vi "SixWheelDriveTrainControl.vi"(0 "dead_or_alive":bool, 1 "Change to Open Loop":bool, 2 "Becky":T1={"DeviceStatus"={"status"=FALSE, "code"=0, "source"=""}, "Type"=enum."PWM", "PWM"={"Digital Module"=enum."Digital Module 1", "PWM Channel"=enum."Invalid", "DeadBand"={"Name"="", "maxPositivePwm"=0, "minPositivePwm"=0, "centerPwm"=0, "maxNegativePwm"=0, "minNegativePwm"=0, "angularRange"=0}}, "CAN"={"Device Number"=0, "Control Mode"=enum."Percent VBus", "Semaphore"=refnum, "Max Vout"=12.0}, "Invert"=FALSE, "TransformRef"=refnum, "InvTransformRef"=refnum}, 3 "Brian":T1={"DeviceStatus"={"status"=FALSE, "code"=0, "source"=""}, "Type"=enum."PWM", "PWM"={"Digital Module"=enum."Digital Module 1", "PWM Channel"=enum."Invalid", "DeadBand"={"Name"="", "maxPositivePwm"=0, "minPositivePwm"=0, "centerPwm"=0, "maxNegativePwm"=0, "minNegativePwm"=0, "angularRange"=0}}, "CAN"={"Device Number"=0, "Control Mode"=enum."Percent VBus", "Semaphore"=refnum, "Max Vout"=12.0}, "Invert"=FALSE, "TransformRef"=refnum, "InvTransformRef"=refnum}, 4 "Curt":T1={"DeviceStatus"={"status"=FALSE, "code"=0, "source"=""}, "Type"=enum."PWM", "PWM"={"Digital Module"=enum."Digital Module 1", "PWM Channel"=enum."Invalid", "DeadBand"={"Name"="", "maxPositivePwm"=0, "minPositivePwm"=0, "centerPwm"=0, "maxNegativePwm"=0, "minNegativePwm"=0, "angularRange"=0}}, "CAN"={"Device Number"=0, "Control Mode"=enum."Percent VBus", "Semaphore"=refnum, "Max Vout"=12.0}, "Invert"=FALSE, "TransformRef"=refnum, "InvTransformRef"=refnum}, 5 "Owen":T1={"DeviceStatus"={"status"=FALSE, "code"=0, "source"=""}, "Type"=enum."PWM", "PWM"={"Digital Module"=enum."Digital Module 1", "PWM Channel"=enum."Invalid", "DeadBand"={"Name"="", "maxPositivePwm"=0, "minPositivePwm"=0, "centerPwm"=0, "maxNegativePwm"=0, "minNegativePwm"=0, "angularRange"=0}}, "CAN"={"Device Number"=0, "Control Mode"=enum."Percent VBus", "Semaphore"=refnum, "Max Vout"=12.0}, "Invert"=FALSE, "TransformRef"=refnum, "InvTransformRef"=refnum}, 6 "CaseVar":i32, 8 "x axis value":dbl, 10 "y axis value":dbl) -> (7 "CaseVarReturn":i32, 9 "x axis value 2":dbl, 11 "y axis value 2":dbl, 16 "BeckyOutput":T1={"DeviceStatus"={"status"=FALSE, "code"=0, "source"=""}, "Type"=enum."PWM", "PWM"={"Digital Module"=enum."Digital Module 1", "PWM Channel"=enum."Invalid", "DeadBand"={"Name"="", "maxPositivePwm"=0, "minPositivePwm"=0, "centerPwm"=0, "maxNegativePwm"=0, "minNegativePwm"=0, "angularRange"=0}}, "CAN"={"Device Number"=0, "Control Mode"=enum."Percent VBus", "Semaphore"=refnum, "Max Vout"=12.0}, "Invert"=FALSE, "TransformRef"=refnum, "InvTransformRef"=refnum}, 17 "BrianOutput":T1={"DeviceStatus"={"status"=FALSE, "code"=0, "source"=""}, "Type"=enum."PWM", "PWM"={"Digital Module"=enum."Digital Module 1", "PWM Channel"=enum."Invalid", "DeadBand"={"Name"="", "maxPositivePwm"=0, "minPositivePwm"=0, "centerPwm"=0, "maxNegativePwm"=0, "minNegativePwm"=0, "angularRange"=0}}, "CAN"={"Device Number"=0, "Control Mode"=enum."Percent VBus", "Semaphore"=refnum, "Max Vout"=12.0}, "Invert"=FALSE, "TransformRef"=refnum, "InvTransformRef"=refnum}, 18 "CurtOutput":T1={"DeviceStatus"={"status"=FALSE, "code"=0, "source"=""}, "Type"=enum."PWM", "PWM"={"Digital Module"=enum."Digital Module 1", "PWM Channel"=enum."Invalid", "DeadBand"={"Name"="", "maxPositivePwm"=0, "minPositivePwm"=0, "centerPwm"=0, "maxNegativePwm"=0, "minNegativePwm"=0, "angularRange"=0}}, "CAN"={"Device Number"=0, "Control Mode"=enum."Percent VBus", "Semaphore"=refnum, "Max Vout"=12.0}, "Invert"=FALSE, "TransformRef"=refnum, "InvTransformRef"=refnum}, 19 "OwenOutput":T1={"DeviceStatus"={"status"=FALSE, "code"=0, "source"=""}, "Type"=enum."PWM", "PWM"={"Digital Module"=enum."Digital Module 1", "PWM Channel"=enum."Invalid", "DeadBand"={"Name"="", "maxPositivePwm"=0, "minPositivePwm"=0, "centerPwm"=0, "maxNegativePwm"=0, "minNegativePwm"=0, "angularRange"=0}}, "CAN"={"Device Number"=0, "Control Mode"=enum."Percent VBus", "Semaphore"=refnum, "Max Vout"=12.0}, "Invert"=FALSE, "TransformRef"=refnum, "InvTransformRef"=refnum})   [LabVIEW 2012]
uses:
  <vilib>/Rock Robotics/WPI/MotorControl/WPI_MotorControlDeviceRef.ctl
  <vilib>/Rock Robotics/SystemInterfaces/Typedef/FPGA_TypedefDigitalModule.ctl
  <vilib>/Rock Robotics/SystemInterfaces/DIO/FPGA_DIOPWMChannel.ctl
  <vilib>/Rock Robotics/WPI/PWM/WPI_PWMDeadband.ctl
  <vilib>/Rock Robotics/WPI/CAN/Jaguar/SubVIs/WPI_CANJaguar_ControlMode.ctl
  <vilib>/Rock Robotics/WPI/PWM/WPI_PWMTransform_ConPane.ctl
  <vilib>/Rock Robotics/WPI/CAN/Jaguar/SubVIs/WPI_CANJaguar_SpeedReference.ctl
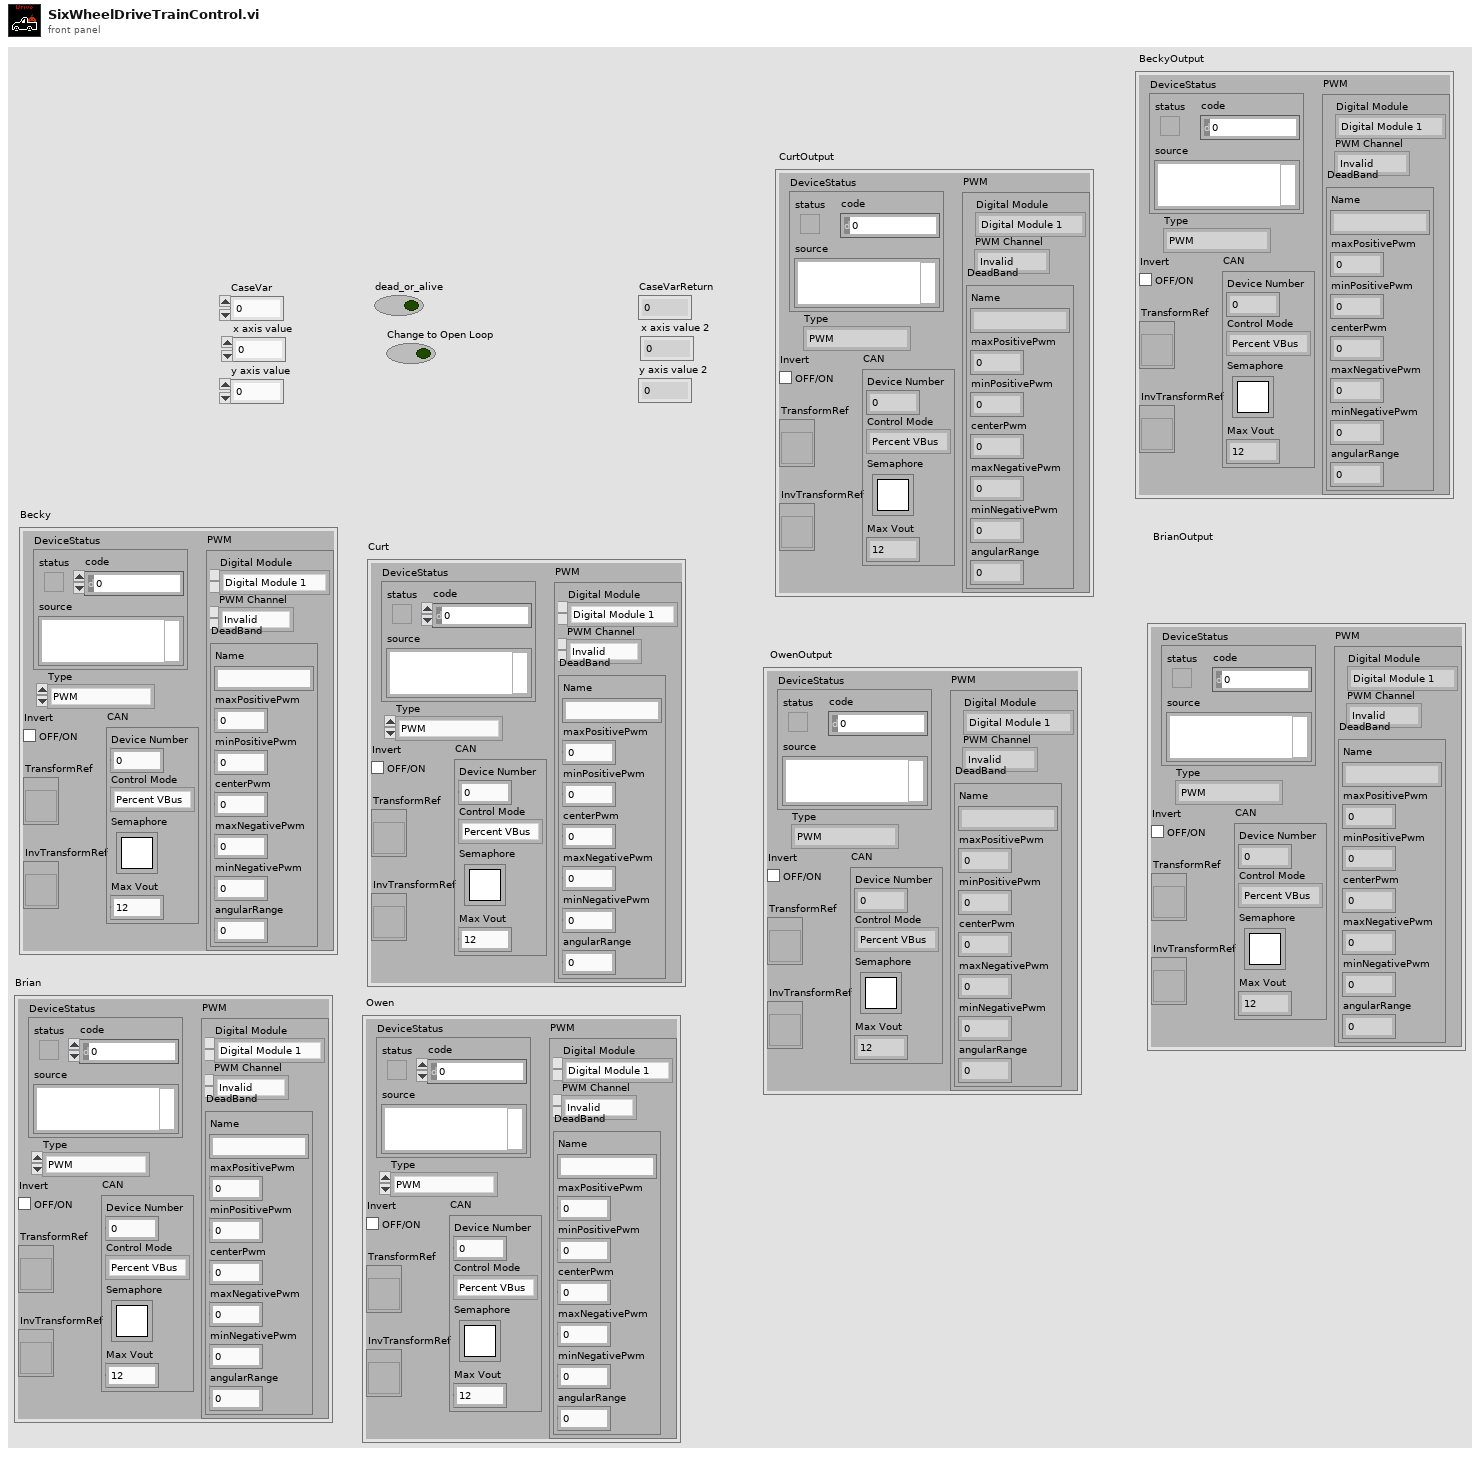
[diagram p1: front panel]
types:
  T1 = typedef "WPI_MotorControlDeviceRef.ctl" = cluster{"DeviceStatus":errorcluster, "Type":enum16{"PWM", "CAN"}, "PWM":cluster{"Digital Module":T2, "PWM Channel":T3, "DeadBand":T4}, "CAN":cluster{"Device Number":u8, "Control Mode":T5, "Semaphore":T6, "Max Vout":dbl}, "Invert":bool, "TransformRef":T7, "InvTransformRef":T7}
  T2 = typedef "FPGA_TypedefDigitalModule.ctl" = enum16{"Digital Module 1", "Digital Module 2"}
  T3 = typedef "FPGA_DIOPWMChannel.ctl" = enum8{"PWM 1", "PWM 2", "PWM 3", "PWM 4", "PWM 5", "PWM 6", "PWM 7", "PWM 8", "PWM 9", "PWM 10", "Invalid"}
  T4 = typedef "WPI_PWMDeadband.ctl" = cluster{"Name":string, "maxPositivePwm":i32, "minPositivePwm":i32, "centerPwm":i32, "maxNegativePwm":i32, "minNegativePwm":i32, "angularRange":u16}
  T5 = typedef "WPI_CANJaguar_ControlMode.ctl" = enum8{"Percent VBus", "Current", "Speed", "Position", "Voltage"}
  T6 = typedef "Semaphore RefNum" = refnum<k1>
  T7 = typedef "WPI_PWMTransform_ConPane.ctl" = refnum<vi>
  T8 = typedef "WPI_CANJaguar_SpeedReference.ctl" = u8
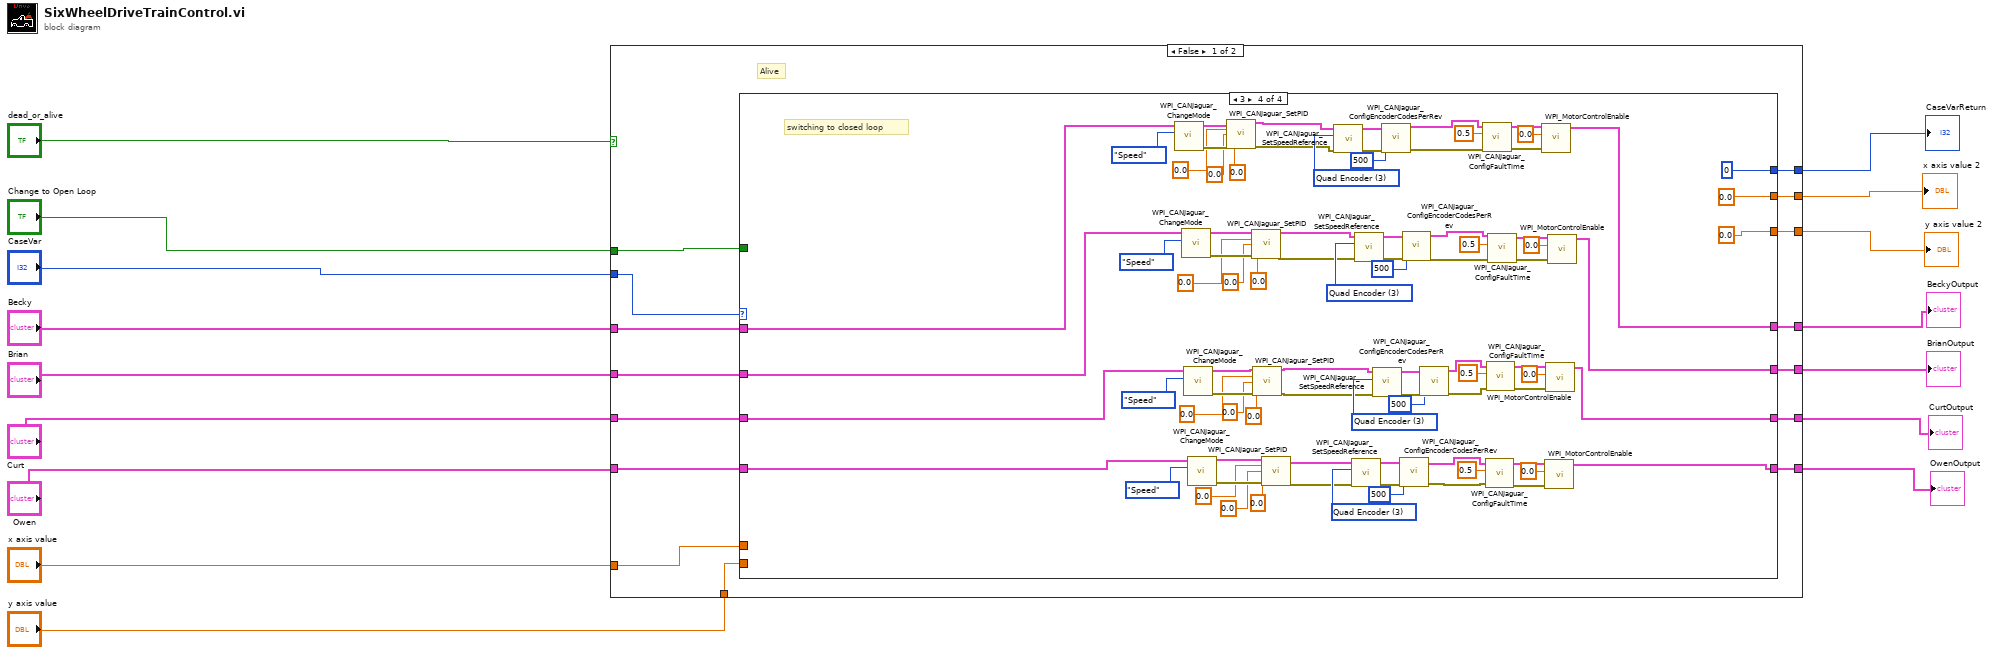
[diagram p0: block diagram]
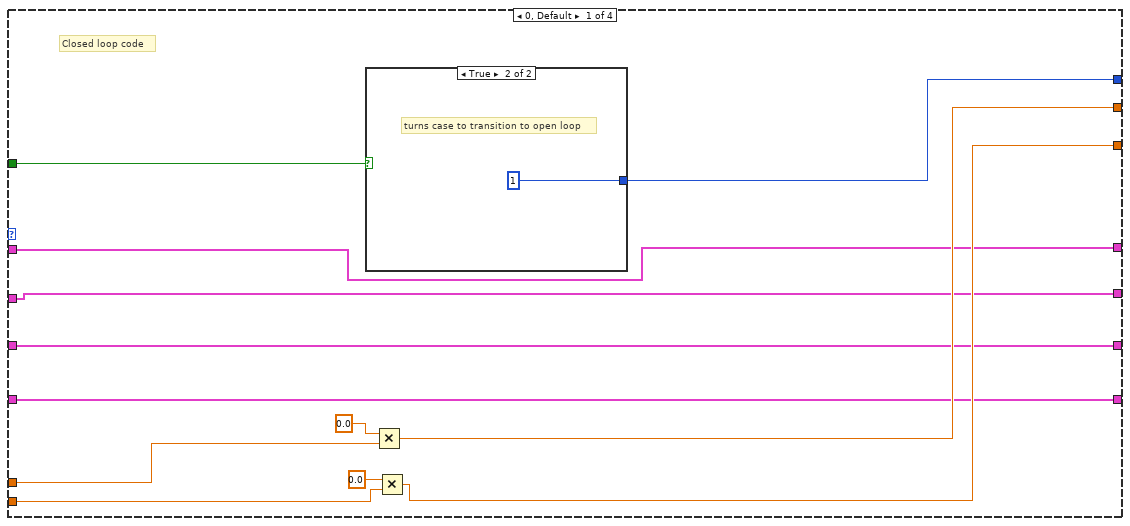
[diagram p2: hidden frame]
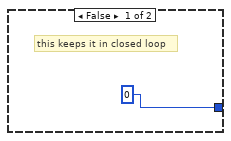
[diagram p3: hidden frame]
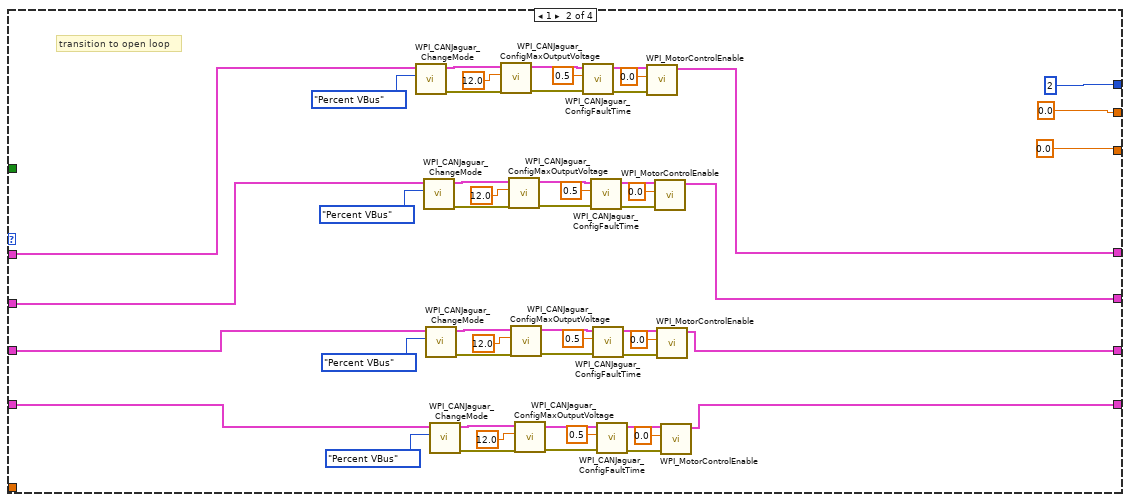
[diagram p4: hidden frame]
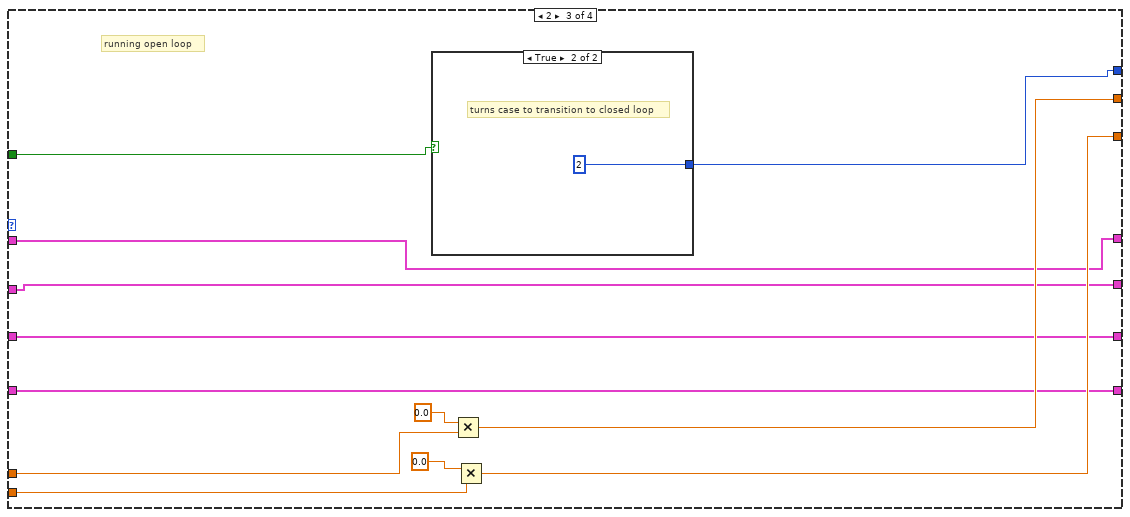
[diagram p5: hidden frame]
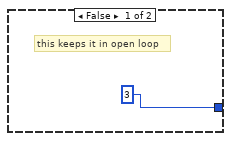
[diagram p6: hidden frame]
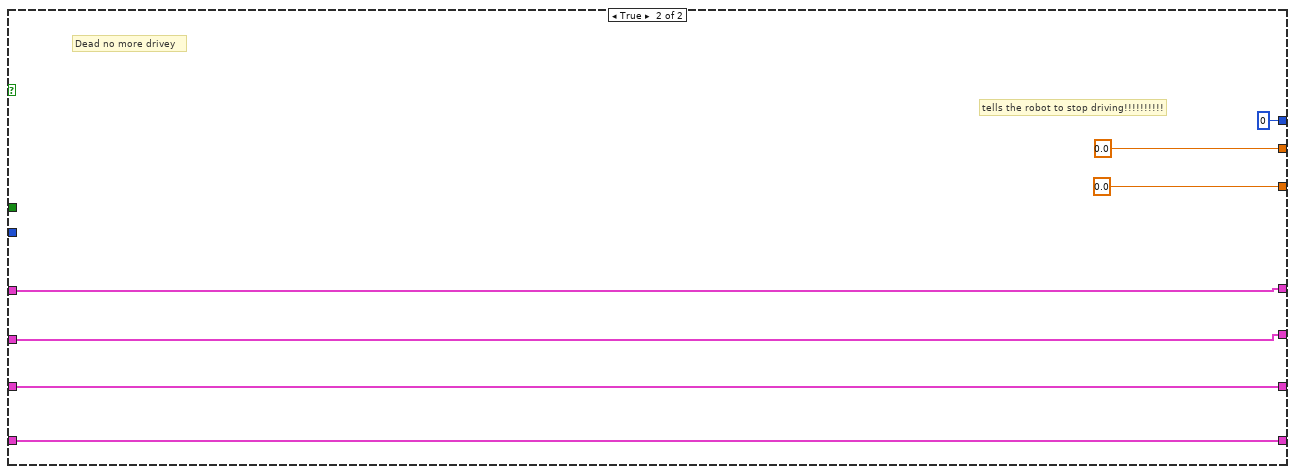
[diagram p7: hidden frame]
diagram:
  n1 = case shown="False" "dead_or_alive" {
    tunnel: [w30 0.0] -> w13
    tunnel: [w29 0.0] -> w12
    tunnel: "CaseVar" -> [w31 _]
    tunnel: [w28 0] -> w14
    tunnel: "Becky" -> [w27 w197]
    tunnel: "Change to Open Loop" -> [w26 _]
    tunnel: "x axis value" -> [w25 _]
    tunnel: "y axis value" -> [w21 _]
    tunnel: "Brian" -> [w24 w196]
    tunnel: "Curt" -> [w23 w195]
    tunnel: "Owen" -> [w22 w194]
    tunnel: [w20 w195] -> w4
    tunnel: [w19 w194] -> w3
    tunnel: [w18 w196] -> w2
    tunnel: [w17 w197] -> w1
    frame False {
      # "Alive"
      n2 = case shown="3" w31 {
        tunnel: w25 -> [w39 _ w104 _]
        tunnel: w21 -> [w38 _ w103 _]
        tunnel: [w36 0.0 w102 0.0] -> w30
        tunnel: [w37 0.0 w101 0.0] -> w29
        tunnel: w26 -> [w43 _ w108 _]
        tunnel: [w42 2 w107 0] -> w28
        tunnel: w27 -> [w32 w54 w97 w173]
        tunnel: w24 -> [w33 w52 w98 w164]
        tunnel: w23 -> [w34 w51 w100 w163]
        tunnel: w22 -> [w35 w50 w99 w162]
        tunnel: [w34 w48 w100 w113] -> w20
        tunnel: [w35 w49 w99 w114] -> w19
        tunnel: [w33 w47 w98 w112] -> w18
        tunnel: [w32 w46 w97 w111] -> w17
        frame 0, Default {
          # "Closed loop code"
          n3 = case shown="True" w43 {
            tunnel: [0 1] -> w42
            frame False {
              # "this keeps it in closed loop"
            }
            frame True {
              # "turns case to transition to open loop"
            }
          }
          n4 = Multiply(x=0.0, y=w39) -> (x*y=w36:dbl)
          n5 = Multiply(x=0.0, y=w38) -> (x*y=w37:dbl)
        }
        frame 1 {
          # "transition to open loop"
          n6 = call <vilib>:"WPI_CANJaguar_ChangeMode.vi"("Control Mode"=WPI_CANJaguar_ControlMode."Percent VBus", "CAN Jaguar Ref"=w54) -> ("error out"=w90:errorcluster, "CAN Jaguar Ref Out"=w93:T1)  [unwired: 8 in]
          n7 = call <vilib>:"WPI_CANJaguar_ChangeMode.vi"("Control Mode"=WPI_CANJaguar_ControlMode."Percent VBus", "CAN Jaguar Ref"=w52) -> ("error out"=w80:errorcluster, "CAN Jaguar Ref Out"=w83:T1)  [unwired: 8 in]
          n8 = call <vilib>:"WPI_CANJaguar_ChangeMode.vi"("Control Mode"=WPI_CANJaguar_ControlMode."Percent VBus", "CAN Jaguar Ref"=w51) -> ("error out"=w62:errorcluster, "CAN Jaguar Ref Out"=w65:T1)  [unwired: 8 in]
          n9 = call <vilib>:"WPI_CANJaguar_ChangeMode.vi"("Control Mode"=WPI_CANJaguar_ControlMode."Percent VBus", "CAN Jaguar Ref"=w50) -> ("error out"=w72:errorcluster, "CAN Jaguar Ref Out"=w55:T1)  [unwired: 8 in]
          n10 = call <vilib>:"WPI_CANJaguar_ConfigMaxOutputVoltage.vi"("error in (no error)"=w90, "Maximum Output Voltage"=12.0, "CAN Jaguar Ref"=w93) -> ("error out"=w89:errorcluster, "CAN Jaguar Ref Out"=w92:T1)  [unwired: 7 in]
          n11 = call <vilib>:"WPI_CANJaguar_ConfigMaxOutputVoltage.vi"("error in (no error)"=w80, "Maximum Output Voltage"=12.0, "CAN Jaguar Ref"=w83) -> ("error out"=w79:errorcluster, "CAN Jaguar Ref Out"=w82:T1)  [unwired: 7 in]
          n12 = call <vilib>:"WPI_CANJaguar_ConfigMaxOutputVoltage.vi"("error in (no error)"=w62, "Maximum Output Voltage"=12.0, "CAN Jaguar Ref"=w65) -> ("error out"=w61:errorcluster, "CAN Jaguar Ref Out"=w64:T1)  [unwired: 7 in]
          n13 = call <vilib>:"WPI_CANJaguar_ConfigMaxOutputVoltage.vi"("error in (no error)"=w72, "Maximum Output Voltage"=12.0, "CAN Jaguar Ref"=w55) -> ("error out"=w71:errorcluster, "CAN Jaguar Ref Out"=w56:T1)  [unwired: 7 in]
          n14 = call <vilib>:"WPI_CANJaguar_ConfigFaultTime.vi"("error in (no error)"=w89, "Fault Time (s)"=0.5, "CAN Jaguar Ref"=w92) -> ("error out"=w88:errorcluster, "CAN Jaguar Ref Out"=w91:T1)  [unwired: 7 in]
          n15 = call <vilib>:"WPI_CANJaguar_ConfigFaultTime.vi"("error in (no error)"=w79, "Fault Time (s)"=0.5, "CAN Jaguar Ref"=w82) -> ("error out"=w78:errorcluster, "CAN Jaguar Ref Out"=w81:T1)  [unwired: 7 in]
          n16 = call <vilib>:"WPI_CANJaguar_ConfigFaultTime.vi"("error in (no error)"=w61, "Fault Time (s)"=0.5, "CAN Jaguar Ref"=w64) -> ("error out"=w60:errorcluster, "CAN Jaguar Ref Out"=w63:T1)  [unwired: 7 in]
          n17 = call <vilib>:"WPI_CANJaguar_ConfigFaultTime.vi"("error in (no error)"=w71, "Fault Time (s)"=0.5, "CAN Jaguar Ref"=w56) -> ("error out"=w70:errorcluster, "CAN Jaguar Ref Out"=w73:T1)  [unwired: 7 in]
          n18 = call <vilib>:"WPI_MotorControlEnable.vi"("error in (no error)"=w88, "Encoder Initial Position"=0.0, "CAN Jaguar Ref"=w91) -> ("CAN Jaguar Ref Out"=w46:T1)  [unwired: 7 in, 1 out]
          n19 = call <vilib>:"WPI_MotorControlEnable.vi"("error in (no error)"=w78, "Encoder Initial Position"=0.0, "CAN Jaguar Ref"=w81) -> ("CAN Jaguar Ref Out"=w47:T1)  [unwired: 7 in, 1 out]
          n20 = call <vilib>:"WPI_MotorControlEnable.vi"("error in (no error)"=w60, "Encoder Initial Position"=0.0, "CAN Jaguar Ref"=w63) -> ("CAN Jaguar Ref Out"=w48:T1)  [unwired: 7 in, 1 out]
          n21 = call <vilib>:"WPI_MotorControlEnable.vi"("error in (no error)"=w70, "Encoder Initial Position"=0.0, "CAN Jaguar Ref"=w73) -> ("CAN Jaguar Ref Out"=w49:T1)  [unwired: 7 in, 1 out]
        }
        frame 2 {
          # "running open loop"
          n22 = case shown="True" w108 {
            tunnel: [3 2] -> w107
            frame False {
              # "this keeps it in open loop"
            }
            frame True {
              # "turns case to transition to closed loop"
            }
          }
          n23 = Multiply(x=0.0, y=w104) -> (x*y=w102:dbl)
          n24 = Multiply(x=0.0, y=w103) -> (x*y=w101:dbl)
        }
        frame 3 {
          w126 = T8 3 items=["Encoder"=0, "Inv Encoder"=2, "Quad Encoder"=3, "None"=255] ("Speed Reference")
          w130 = T8 3 items=["Encoder"=0, "Inv Encoder"=2, "Quad Encoder"=3, "None"=255] ("Speed Reference")
          w138 = T8 3 items=["Encoder"=0, "Inv Encoder"=2, "Quad Encoder"=3, "None"=255] ("Speed Reference")
          w146 = T8 3 items=["Encoder"=0, "Inv Encoder"=2, "Quad Encoder"=3, "None"=255] ("Speed Reference")
          # "switching to closed loop"
          n25 = call <vilib>:"WPI_CANJaguar_ChangeMode.vi"("Control Mode"=WPI_CANJaguar_ControlMode."Speed", "CAN Jaguar Ref"=w173) -> ("error out"=w168:errorcluster, "CAN Jaguar Ref Out"=w169:T1)  [unwired: 8 in]
          n26 = call <vilib>:"WPI_CANJaguar_ChangeMode.vi"("Control Mode"=WPI_CANJaguar_ControlMode."Speed", "CAN Jaguar Ref"=w164) -> ("error out"=w159:errorcluster, "CAN Jaguar Ref Out"=w165:T1)  [unwired: 8 in]
          n27 = call <vilib>:"WPI_CANJaguar_ChangeMode.vi"("Control Mode"=WPI_CANJaguar_ControlMode."Speed", "CAN Jaguar Ref"=w163) -> ("error out"=w160:errorcluster, "CAN Jaguar Ref Out"=w166:T1)  [unwired: 8 in]
          n28 = call <vilib>:"WPI_CANJaguar_ChangeMode.vi"("Control Mode"=WPI_CANJaguar_ControlMode."Speed", "CAN Jaguar Ref"=w162) -> ("error out"=w161:errorcluster, "CAN Jaguar Ref Out"=w167:T1)  [unwired: 8 in]
          n29 = call <vilib>:"WPI_CANJaguar_SetPID.vi"("CAN Jaguar Ref"=w169, "P"=0.0, "I"=0.0, "D"=0.0, "error in (no error)"=w168) -> ("CAN Jaguar Ref Out"=w119:T1, "error out"=w122:errorcluster)  [unwired: 9 in]
          n30 = call <vilib>:"WPI_CANJaguar_SetPID.vi"("CAN Jaguar Ref"=w165, "P"=0.0, "I"=0.0, "D"=0.0, "error in (no error)"=w159) -> ("CAN Jaguar Ref Out"=w142:T1, "error out"=w139:errorcluster)  [unwired: 9 in]
          n31 = call <vilib>:"WPI_CANJaguar_SetPID.vi"("CAN Jaguar Ref"=w166, "P"=0.0, "I"=0.0, "D"=0.0, "error in (no error)"=w160) -> ("CAN Jaguar Ref Out"=w134:T1, "error out"=w133:errorcluster)  [unwired: 9 in]
          n32 = call <vilib>:"WPI_CANJaguar_SetPID.vi"("CAN Jaguar Ref"=w167, "P"=0.0, "I"=0.0, "D"=0.0, "error in (no error)"=w161) -> ("CAN Jaguar Ref Out"=w116:T1, "error out"=w115:errorcluster)  [unwired: 9 in]
          n33 = call <vilib>:"WPI_CANJaguar_SetSpeedReference.vi"("error in (no error)"=w122, "Speed Reference"=w126, "CAN Jaguar Ref"=w119) -> ("error out"=w125:errorcluster, "CAN Jaguar Ref Out"=w124:T1)  [unwired: 7 in]
          n34 = call <vilib>:"WPI_CANJaguar_SetSpeedReference.vi"("error in (no error)"=w115, "Speed Reference"=w130, "CAN Jaguar Ref"=w116) -> ("error out"=w129:errorcluster, "CAN Jaguar Ref Out"=w128:T1)  [unwired: 7 in]
          n35 = call <vilib>:"WPI_CANJaguar_SetSpeedReference.vi"("error in (no error)"=w139, "Speed Reference"=w146, "CAN Jaguar Ref"=w142) -> ("error out"=w145:errorcluster, "CAN Jaguar Ref Out"=w144:T1)  [unwired: 7 in]
          n36 = call <vilib>:"WPI_CANJaguar_SetSpeedReference.vi"("error in (no error)"=w133, "Speed Reference"=w138, "CAN Jaguar Ref"=w134) -> ("error out"=w137:errorcluster, "CAN Jaguar Ref Out"=w136:T1)  [unwired: 7 in]
          n37 = call <vilib>:"WPI_CANJaguar_ConfigEncoderCodesPerRev.vi"("error in (no error)"=w125, "Encoder Codes Per Rev"=u16 500, "CAN Jaguar Ref"=w124) -> ("error out"=w121:errorcluster, "CAN Jaguar Ref Out"=w120:T1)  [unwired: 7 in]
          n38 = call <vilib>:"WPI_CANJaguar_ConfigEncoderCodesPerRev.vi"("error in (no error)"=w129, "Encoder Codes Per Rev"=u16 500, "CAN Jaguar Ref"=w128) -> ("error out"=w118:errorcluster, "CAN Jaguar Ref Out"=w117:T1)  [unwired: 7 in]
          n39 = call <vilib>:"WPI_CANJaguar_ConfigEncoderCodesPerRev.vi"("error in (no error)"=w145, "Encoder Codes Per Rev"=u16 500, "CAN Jaguar Ref"=w144) -> ("error out"=w140:errorcluster, "CAN Jaguar Ref Out"=w141:T1)  [unwired: 7 in]
          n40 = call <vilib>:"WPI_CANJaguar_ConfigEncoderCodesPerRev.vi"("error in (no error)"=w137, "Encoder Codes Per Rev"=u16 500, "CAN Jaguar Ref"=w136) -> ("error out"=w131:errorcluster, "CAN Jaguar Ref Out"=w132:T1)  [unwired: 7 in]
          n41 = call <vilib>:"WPI_CANJaguar_ConfigFaultTime.vi"("error in (no error)"=w121, "Fault Time (s)"=0.5, "CAN Jaguar Ref"=w120) -> ("error out"=w191:errorcluster, "CAN Jaguar Ref Out"=w192:T1)  [unwired: 7 in]
          n42 = call <vilib>:"WPI_CANJaguar_ConfigFaultTime.vi"("error in (no error)"=w118, "Fault Time (s)"=0.5, "CAN Jaguar Ref"=w117) -> ("error out"=w181:errorcluster, "CAN Jaguar Ref Out"=w182:T1)  [unwired: 7 in]
          n43 = call <vilib>:"WPI_CANJaguar_ConfigFaultTime.vi"("error in (no error)"=w131, "Fault Time (s)"=0.5, "CAN Jaguar Ref"=w132) -> ("error out"=w176:errorcluster, "CAN Jaguar Ref Out"=w177:T1)  [unwired: 7 in]
          n44 = call <vilib>:"WPI_CANJaguar_ConfigFaultTime.vi"("error in (no error)"=w140, "Fault Time (s)"=0.5, "CAN Jaguar Ref"=w141) -> ("error out"=w186:errorcluster, "CAN Jaguar Ref Out"=w187:T1)  [unwired: 7 in]
          n45 = call <vilib>:"WPI_MotorControlEnable.vi"("error in (no error)"=w191, "Encoder Initial Position"=0.0, "CAN Jaguar Ref"=w192) -> ("CAN Jaguar Ref Out"=w111:T1)  [unwired: 7 in, 1 out]
          n46 = call <vilib>:"WPI_MotorControlEnable.vi"("error in (no error)"=w181, "Encoder Initial Position"=0.0, "CAN Jaguar Ref"=w182) -> ("CAN Jaguar Ref Out"=w114:T1)  [unwired: 7 in, 1 out]
          n47 = call <vilib>:"WPI_MotorControlEnable.vi"("error in (no error)"=w176, "Encoder Initial Position"=0.0, "CAN Jaguar Ref"=w177) -> ("CAN Jaguar Ref Out"=w113:T1)  [unwired: 7 in, 1 out]
          n48 = call <vilib>:"WPI_MotorControlEnable.vi"("error in (no error)"=w186, "Encoder Initial Position"=0.0, "CAN Jaguar Ref"=w187) -> ("CAN Jaguar Ref Out"=w112:T1)  [unwired: 7 in, 1 out]
        }
      }
    }
    frame True {
      # "Dead no more drivey"
      # "tells the robot to stop driving!!!!!!!!!!"
    }
  }
  "CaseVarReturn" <- w14
  "x axis value 2" <- w13
  "y axis value 2" <- w12
  "OwenOutput" <- w3
  "CurtOutput" <- w4
  "BeckyOutput" <- w1
  "BrianOutput" <- w2
